vi "sample_from_gaussian.vi"(10 "standard deviation":dbl=1.0 format="%0.2f", 11 "Samples":i32) -> (3 "Output":dbl[](array[numeric]))   [LabVIEW 2019]
uses:
  <vilib>/ptbypt/NI_PtbyPt.lvlib
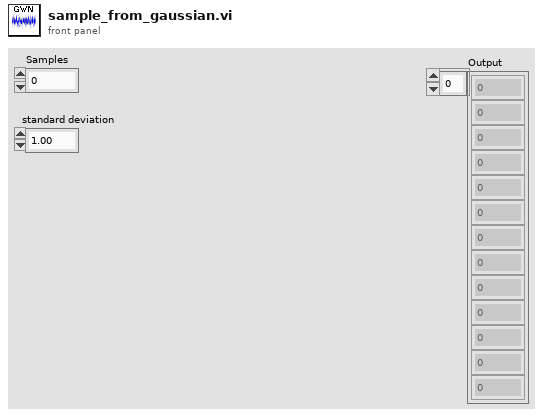
[diagram p1: front panel]
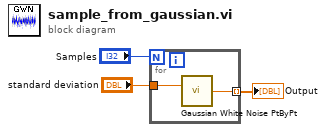
[diagram p0: block diagram]
diagram:
  n1 = for {
    N: "Samples" -> [_]
    tunnel: "standard deviation" -> [w5]
    tunnel: [w4] -> w1 mode=indexing
    n2 = call <vilib>:"Gaussian White Noise PtByPt.vi"("standard deviation"=w5) -> ("Gaussian white noise"=w4:dbl)  [unwired: 2 in]
  }
  "Output" <- w1
